vi "ArrayRead_S.vi"(0 "Current (or Cued Trial Parameters)":string[](array[string])) -> (4 "Value 0":string, 6 "Value 1":string, 8 "Value 2":string, 10 "Value 3":string, 11 "Value 8":string, 12 "Value 7":string, 13 "Value 6":string, 14 "Value 5":string, 15 "Value 4":string)   [LabVIEW 2009]
doc: "This VI allows you to access the first 9 elements in a double array. If there are less elements, you will get the default value of zero in return."
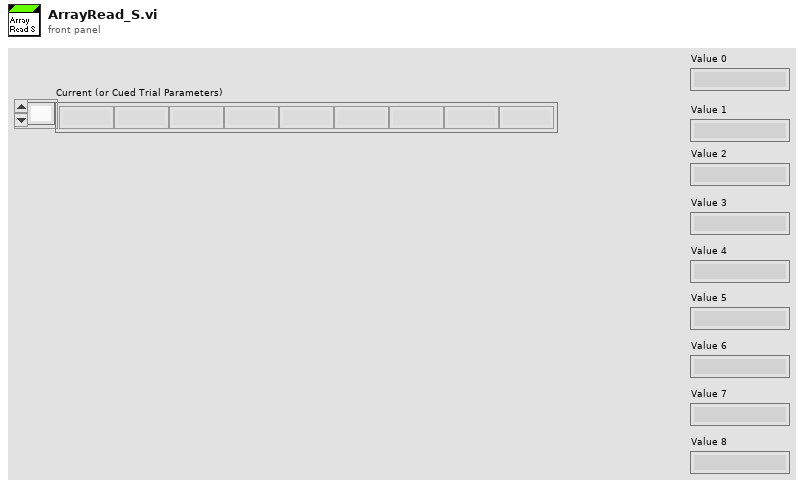
[diagram p1: front panel]
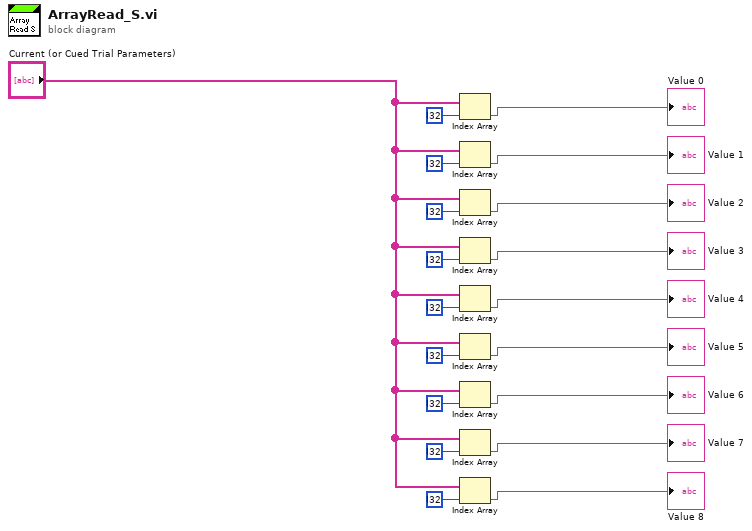
[diagram p0: block diagram]
diagram:
  n1 = Index Array(array="Current (or Cued Trial Parameters)", index=i32 ?) -> (element=→"Value 0":string)
  n2 = Index Array(array="Current (or Cued Trial Parameters)", index=i32 ?) -> (element=→"Value 1":string)
  n3 = Index Array(array="Current (or Cued Trial Parameters)", index=i32 ?) -> (element=→"Value 2":string)
  n4 = Index Array(array="Current (or Cued Trial Parameters)", index=i32 ?) -> (element=→"Value 3":string)
  n5 = Index Array(array="Current (or Cued Trial Parameters)", index=i32 ?) -> (element=→"Value 4":string)
  n6 = Index Array(array="Current (or Cued Trial Parameters)", index=i32 ?) -> (element=→"Value 5":string)
  n7 = Index Array(array="Current (or Cued Trial Parameters)", index=i32 ?) -> (element=→"Value 6":string)
  n8 = Index Array(array="Current (or Cued Trial Parameters)", index=i32 ?) -> (element=→"Value 7":string)
  n9 = Index Array(array="Current (or Cued Trial Parameters)", index=i32 ?) -> (element=→"Value 8":string)
